vi "rs3 init disparity_to_depth.vi"(8 "error in (no error)":errorcluster) -> (0 "error out":errorcluster, 1 "error frame queue":u64, 2 "error disp transf block":u64, 3 "error start processing":u64, 4 "disparity_transforg_2_block":u64, 5 "disparity transforg_2_queue":u64)   [LabVIEW 2017, in "libRealSense3.lvlib"]
doc: "This initialized the processing block & queue to be able to transform from disparity space to depth (z=1/D)."
uses:
  libRealSense3.lvlib
panel:
  # "RS3 Init Disparity-To-Depth"
  # "(C) Intel Corp.,  AGJ"
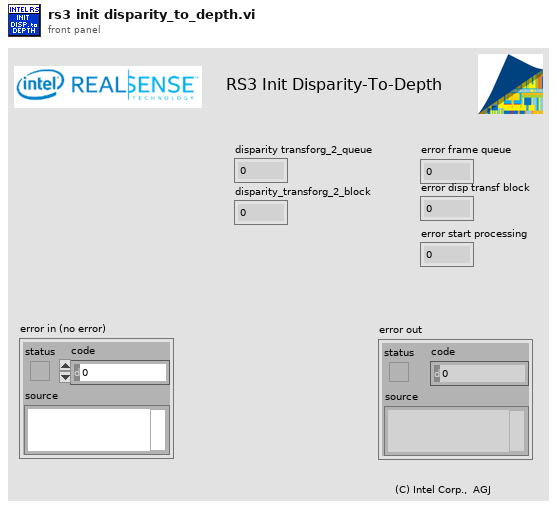
[diagram p1: front panel]
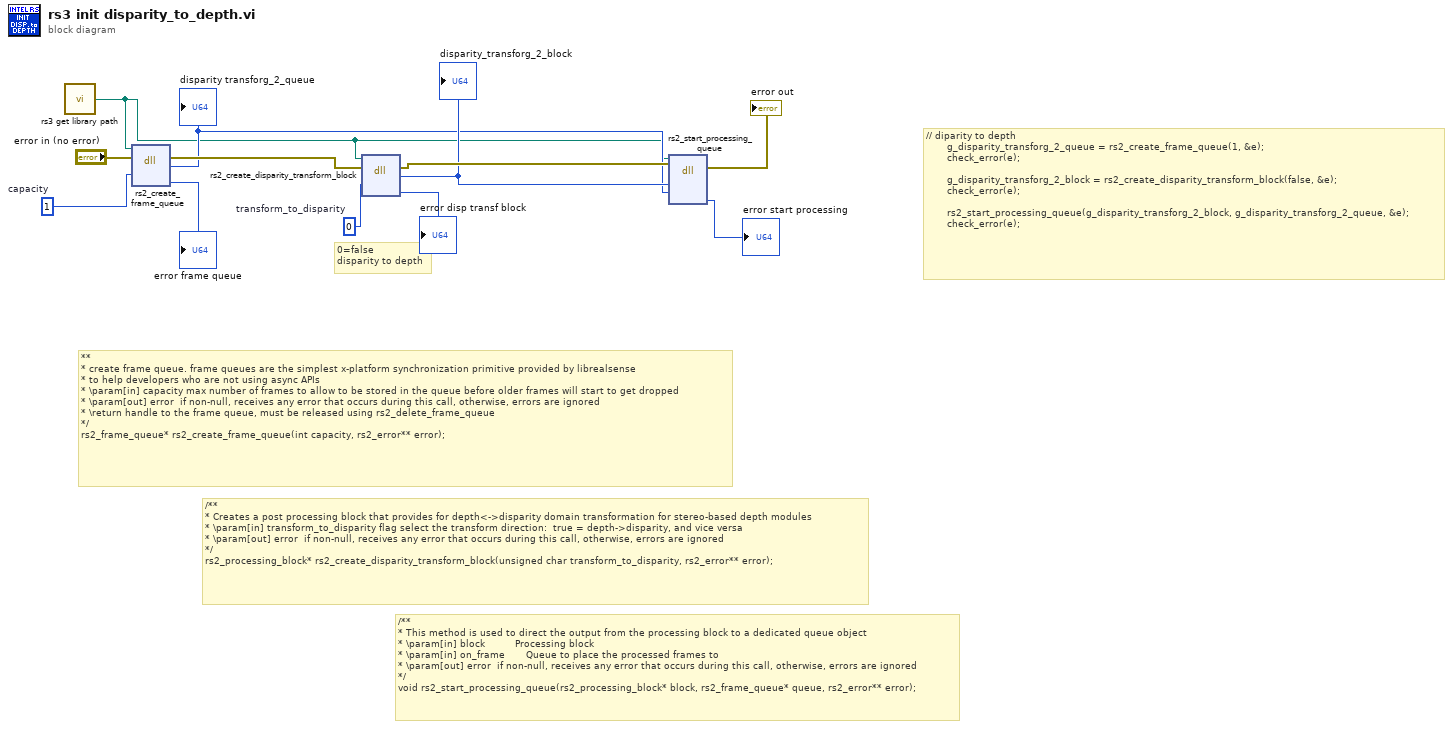
[diagram p0: block diagram]
diagram:
  w11 = 1  # capacity
  w2 = u8 0  # transform_to_disparity
  # "0=false \ndisparity to depth"
  # "/**\n* Creates a post processing block that provides for depth<->disparity domain transformation for stereo-based depth modules\n* \\param[in] transform_to_disparity flag select the transform direction:  true = depth->disparity, and vice versa\n* \\param[out] error  if non-null, receives any error that occurs during this call, otherwise, errors are ignored\n*/\nrs2_processing_block* rs2_create_disparity_transform_block(unsigned char transform_to_disparity, rs2_error** error);"
  # "// diparity to depth\n       g_disparity_transforg_2_queue = rs2_create_frame_queue(1, &e);\n       check_error(e);\n\n       g_disparity_transforg_2_block = rs2_create_disparity_transform_block(false, &e);\n       check_error(e);\n\n       rs2_start_processing_queue(g_disparity_transforg_2_block, g_disparity_transforg_2_queue, &e);\n       check_error(e);"
  # "/**\n* This method is used to direct the output from the processing block to a dedicated queue object\n* \\param[in] block          Processing block\n* \\param[in] on_frame       Queue to place the processed frames to\n* \\param[out] error  if non-null, receives any error that occurs during this call, otherwise, errors are ignored\n*/\nvoid rs2_start_processing_queue(rs2_processing_block* block, rs2_frame_queue* queue, rs2_error** error);"
  # "**\n* create frame queue. frame queues are the simplest x-platform synchronization primitive provided by librealsense\n* to help developers who are not using async APIs\n* \\param[in] capacity max number of frames to allow to be stored in the queue before older frames will start to get dropped\n* \\param[out] error  if non-null, receives any error that occurs during this call, otherwise, errors are ignored\n* \\return handle to the frame queue, must be released using rs2_delete_frame_queue\n*/\nrs2_frame_queue* rs2_create_frame_queue(int capacity, rs2_error** error);"
  n1 = call "rs3 get library path.vi"() -> ("Realsense 2 Library Path"=w1:path)
  n2 = dll-call lib="C:/Users/agrunnet/Documents/libRealSense6/realsense2.dll" fn="rs2_create_frame_queue"(path in=w1, error in="error in (no error)", "capacity"=w11) -> (error out=w9:errorcluster, "decimation filter queue"=w4:u64, "error"=→"error frame queue":u64)  [unwired: 3 in, 1 out]
  "disparity transforg_2_queue" <- w4
  n3 = dll-call lib="C:/Users/agrunnet/Documents/libRealSense6/realsense2.dll" fn="rs2_create_disparity_transform_block"(path in=w1, error in=w9, "transform_to_disparity"=w2) -> (error out=w7:errorcluster, "disparity_transform_1_block"=w5:u64, "error"=→"error disp transf block":u64)  [unwired: 3 in, 1 out]
  "disparity_transforg_2_block" <- w5
  n4 = dll-call lib="C:/Users/agrunnet/Documents/libRealSense6/realsense2.dll" fn="rs2_start_processing_queue"(path in=w1, error in=w7, "processing block"=w5, "frame queue"=w4) -> (error out=→"error out":errorcluster, "error"=→"error start processing":u64)  [unwired: 5 in, 1 out]
